vi "starSystemControl.vi"() -> ()   [LabVIEW 2021]
doc: "This example demonstrates how to call a Python function and pass doubles as arguments. It uses a python function to compute the sum of two doubles."
uses:
  <extravilib>/ChannelInstances/Tag-bool/Write With Abort.vi
  <extravilib>/ChannelInstances/Tag-bool/Read With Abort.vi
  <extravilib>/ChannelInstances/Tag-bool/Instantiate.vi
  <extravilib>/ChannelInstances/Tag-bool/EndpointRead.vi
  globalVariables.vi
  <extravilib>/ChannelInstances/Tag-bool/Endpoint.vi
  <extravilib>/ChannelInstances/Tag-bool.lvlib
  Copy of Kloehn V6 Series Folder/Copy of Kloehn V6 Series.lvlib
panel:
  out "armError":errorcluster
  in  "Motion":T1={"Top Speed (5000 sps) "=3000, "Start Speed (750 sps)"=750, "Stop Speed (750 sps)"=750, "Accel (17500 st/s^2)"=17500, "Decel (17500 st/s^2)"=17500, "Backlash Steps (100 steps)"=100}
  in  "syringeTotalVol":dbl=2.5
  in  "cDAQDirection_p1":tag="cDAQ1Mod1/port0/line0"
  in  "cDAQVoltage_p1":tag="cDAQ1Mod2/ao0"
  in  "voltage_p1":dbl=1.2 format="%#_3g"
  in  "rate_p1":dbl=2.6 format="%#_3g"
  in  "cDAQDirection_p2":tag="cDAQ1Mod1/port0/line1"
  in  "cDAQVoltage_p2":tag="cDAQ1Mod2/ao1"
  in  "locationPythonCode":path=path "C:/Users/coralProgram/Documents/armand/xArm-Python-SDK-master/main.py"
  in  "pythonVersion":dbl=3.9
  in  "robotName":string="a1"
  in  "pumpReverseVol":dbl=0.2
  in  "syringeReverseVol":dbl=0.2
  in  "voltage_p2":dbl=1.24 format="%#_3g"
  in  "rate_p2":dbl=2.09 caption="rate_p1" format="%#_3g"
  out "syringeError":errorcluster
  out "Response":string
  out "commandString":string
  in  "VISA Refnum in":refnum<visa-resource-name>="COM8"
  out "Gauge":dbl(knob) scale=0.0..7.0
  out "syringeState":dbl(slide)
  out "Position":dbl
  out "Busy":bool
  in  "Serial Configuration":cluster{"Baud Rate":u32, "Address":u16}={"Baud Rate"=9600, "Address"=1} {"Address" max=15 step=1}
  in  "VISA resource name":refnum<visa-resource-name>="COM7"
  in  "Array":dbl[][](array[numeric])=[[0.0, 10.0, 1.0], [10.0, 0.0, 1.0], [0.0, 10.0, 1.0], [10.0, 0.0, 1.0], [0.0, 10.0, 1.0], [10.0, 0.0, 1.0], [0.0, 10.0, 1.0], [10.0, 0.0, 1.0], [0.0, 10.0, 1.0], [10.0, 0.0, 1.0], [0.0, 10.0, 1.0], [10.0, 0.0, 1.0], [0.0, 10.0, 1.0], [10.0, 0.0, 1.0], [0.0, 10.0, 1.0], [10.0, 0.0, 1.0], [0.0, 10.0, 1.0], [10.0, 0.0, 1.0], [0.0, 10.0, 1.0], [10.0, 0.0, 1.0], [0.0, 10.0, 1.0], [10.0, 0.0, 1.0], [0.0, 10.0, 1.0], [10.0, 0.0, 1.0], [0.0, 10.0, 1.0], [10.0, 0.0, 1.0], [0.0, 10.0, 1.0], [10.0, 0.0, 1.0], [0.0, 10.0, 1.0], [10.0, 0.0, 1.0], [0.0, 10.0, 1.0], [10.0, 0.0, 1.0], [0.0, 10.0, 1.0], [10.0, 0.0, 1.0], [0.0, 10.0, 1.0], [10.0, 0.0, 1.0], [0.0, 10.0, 1.0], [10.0, 0.0, 1.0], [0.0, 10.0, 1.0], [10.0, 0.0, 1.0], [0.0, 10.0, 1.0], [10.0, 0.0, 1.0], [0.0, 10.0, 1.0], [10.0, 0.0, 1.0], [0.0, 10.0, 1.0], [10.0, 0.0, 1.0], [0.0, 10.0, 1.0], [10.0, 0.0, 1.0]]
  in  "stop_p1":bool caption="stop"
  out "position":dbl=45.0
  # "STAR System"
  # "Name"
  # "T1"
  # "Arm"
  # "Position"
  # "T2"
  # "T3"
  # "Python code location"
  # "Version"
  # "T4"
  # "T5"
  # "T6"
  # "Watchdog"
  # "Syringe error"
  # "T7"
  # "T8"
  # "Port"
  # "T9"
  # "T10"
  # "T11"
  # "Arm error"
  # "Command"
  # "T12"
  # "T13"
  # "Response"
  # "T14"
  # "T15"
  # "T16"
  # "T17"
  # "Syringe"
  # "T18"
  # "T19"
  # "Port"
  # "T20"
  # "Baud"
  # "T21"
  # "T22"
  # "Address"
  # "T23"
  # "T24"
  # "Total vol (mL)"
  # "T25"
  # "Reverse (mL)"
  # "T26"
  # "T27"
  # "Position"
  # "Busy"
  # "T28"
  # "T29"
  # "T30"
  # "T31"
  # "T32"
  # "T33"
  # "T34"
  # "T35"
  # "T36"
  # "T37"
  # "Pumps"
  # "Reverse (mL)"
  # "T38"
  # "T39"
  # "Pump 1"
  # "Pump 2"
  # "T40"
  # "Voltage"
  # "T41"
  # "T42"
  # "Rate (mL/S)"
  # "T43"
  # "T44"
  # "Voltage address"
  # "T45"
  # "T46"
  # "Direction address"
  # "T47"
  # "T48"
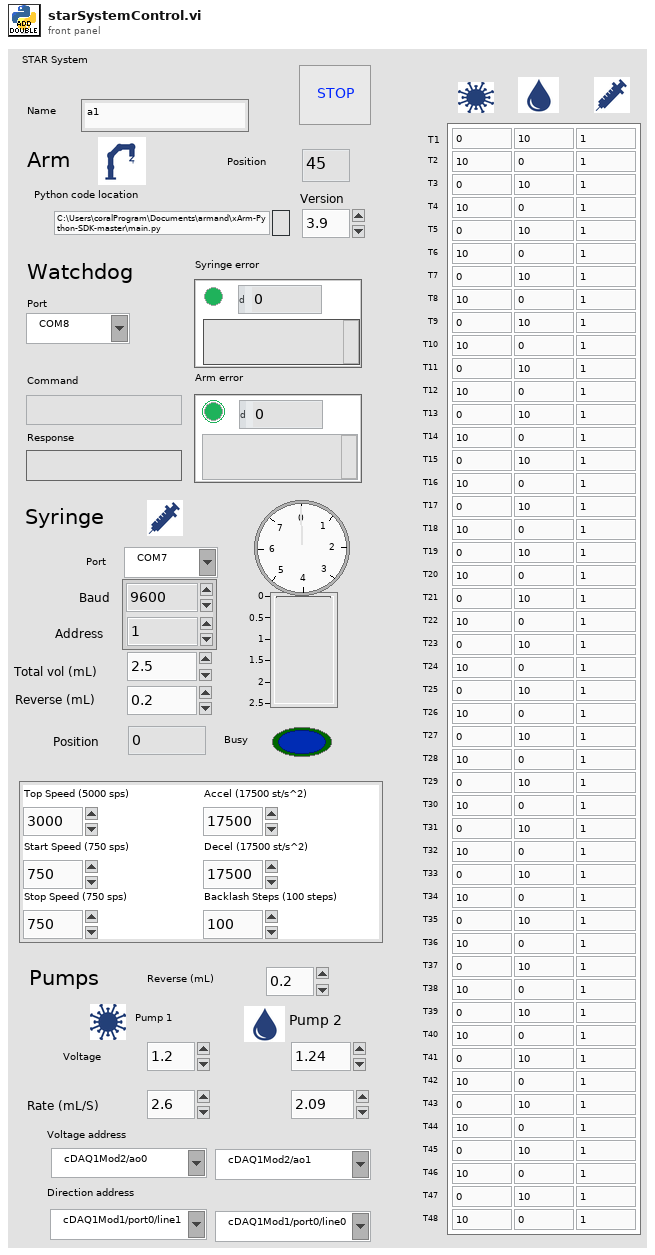
[diagram p1: front panel]
types:
  T1 = cluster{"Top Speed (5000 sps) ":i32, "Start Speed (750 sps)":i32, "Stop Speed (750 sps)":i32, "Accel (17500 st/s^2)":i32, "Decel (17500 st/s^2)":i32, "Backlash Steps (100 steps)":i32}
  T2 = typedef "Tag-bool.lvlib/))Channel.ctl" = refnum<queue>
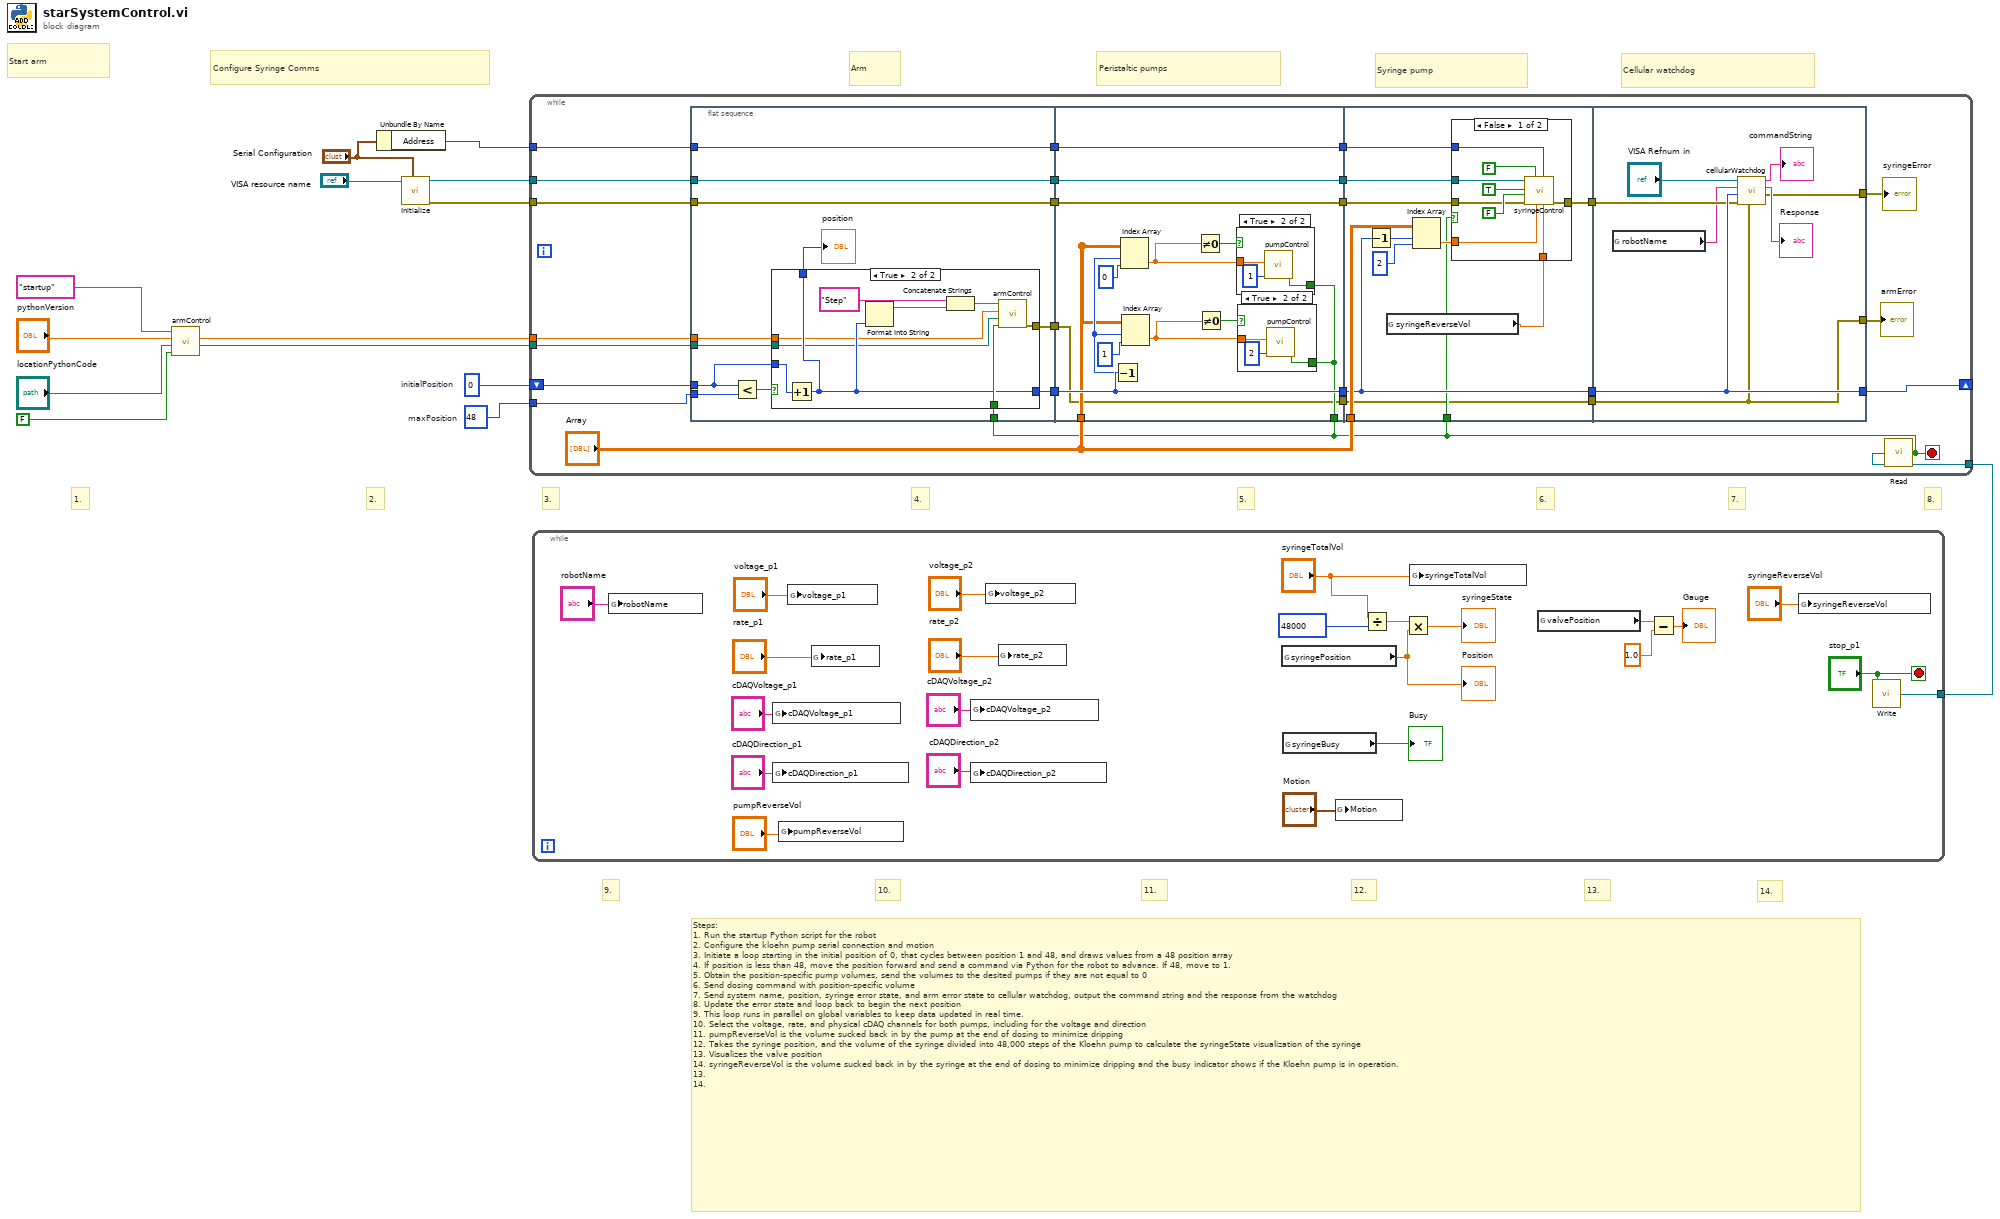
[diagram p0: block diagram]
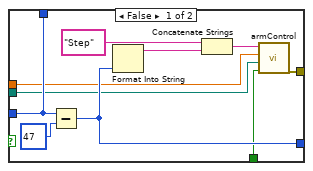
[diagram p2: hidden frame]
diagram:
  w12 = 48  # maxPosition
  w14 = 0  # initialPosition
  # "Start arm"
  # "Cellular watchdog"
  # "Syringe pump"
  # "Peristaltic pumps"
  # "Arm"
  # "14."
  # "Steps:\n1. Run the startup Python script for the robot\n2. Configure the kloehn pump serial connection and motion\n3. Initiate a loop starting in the initial position of 0, that cycles between position 1 and 48, and draws values from a 48 position array \n4. If position is less than 48, move the position forward and send a command via Python for the robot to advance. If 48, move to 1. \n5. Obtain the position-specific pump volumes, send the volumes to the desited pumps if they are not equal to 0\n6. Send dosing command with position-specific volume\n7. Send system name, position, syringe error state, and arm error state to cellular watchdog, output the command string and the response from the watchdog\n8. Update the error state and loop back to begin the next position\n9. This loop runs in parallel on global variables to keep data updated in real time. \n10. Select the voltage, rate, and physical cDAQ channels for both pumps, including for the voltage and direction\n11. pumpReverseVol is the volume sucked back in by the pump at the end of dosing to minimize dripping\n12. Takes the syringe position, and the volume of the syringe divided into 48,000 steps of the Kloehn pump to calculate the syringeState visualization of the syringe\n13. Visualizes the valve position\n14. syringeReverseVol is the volume sucked back in by the syringe at the end of dosing to minimize dripping and the busy indicator shows if the Kloehn pump is in operation.\n13.\n14."
  # "13."
  # "12."
  # "11."
  # "1."
  # "9."
  # "10."
  # "7."
  # "6."
  # "5."
  # "4."
  # "3."
  # "2."
  # "8."
  # "Configure Syringe Comms"
  n1 = call "armControl.vi"("Off"=FALSE ("buttonRefill"), "locationPythonCode"="locationPythonCode", "pythonVersionIn"="pythonVersion", "commandInput"="startup") -> ("locationPythonCodeOutput"=w3:path, "pythonVersionOut"=w4:dbl)  [unwired: 3 in, 2 out]
  n2 = Unbundle By Name("Serial Configuration") -> ("Address"=w6:u16)
  n3 = call "Initialize.vi"("Serial Configuration"="Serial Configuration", "VISA resource name"="VISA resource name") -> ("error out"=w8:errorcluster, "VISA resource name out"=w7:refnum<visa-resource-name>)  [unwired: 8 in]
  n4 = while {
    tunnel: [w37] -> w13
    stop <- "stop_p1" stop-if-true
    n5 = global write "globalVariables.vi" "robotName"("robotName") -> ()
    n6 = global write "globalVariables.vi" "cDAQVoltage_p1"("cDAQVoltage_p1") -> ()
    n7 = global write "globalVariables.vi" "cDAQDirection_p1"("cDAQDirection_p1") -> ()
    n8 = global write "globalVariables.vi" "pumpReverseVol"("pumpReverseVol") -> ()
    n9 = global write "globalVariables.vi" "voltage_p1"("voltage_p1") -> ()
    n10 = global write "globalVariables.vi" "rate_p1"("rate_p1") -> ()
    n11 = global write "globalVariables.vi" "cDAQVoltage_p2"("cDAQVoltage_p2") -> ()
    n12 = global write "globalVariables.vi" "cDAQDirection_p2"("cDAQDirection_p2") -> ()
    n13 = global write "globalVariables.vi" "voltage_p2"("voltage_p2") -> ()
    n14 = global write "globalVariables.vi" "rate_p2"("rate_p2") -> ()
    n15 = global read "globalVariables.vi" "syringePosition"() -> (w27:dbl)
    "Position" <- w27
    n16 = global read "globalVariables.vi" "syringeBusy"() -> (→"Busy":bool)
    n17 = global write "globalVariables.vi" "Motion"("Motion") -> ()
    n18 = Divide(x="syringeTotalVol", y=48000) -> (x/y=w34:dbl)
    n19 = Multiply(x=w34, y=w27) -> (x*y=→"syringeState":dbl)
    n20 = global write "globalVariables.vi" "syringeTotalVol"("syringeTotalVol") -> ()
    n21 = global read "globalVariables.vi" "valvePosition"() -> (w26:dbl)
    n22 = Subtract(x=w26, y=1.0) -> (x-y=→"Gauge":dbl)
    n23 = global write "globalVariables.vi" "syringeReverseVol"("syringeReverseVol") -> ()
    n24 = call <extravilib>:"Write.vi"("element"="stop_p1") -> ("channel"=w37:T2)  [unwired: 1 out]
  }
  n25 = while {
    shift-right: [w61] -> _
    shift-left: w14 -> [w44]
    tunnel: w13 -> [w63]
    tunnel: w12 -> [w62]
    tunnel: w8 -> [w59]
    tunnel: w7 -> [w48]
    tunnel: w6 -> [w47]
    tunnel: w4 -> [w43]
    tunnel: w3 -> [w42]
    stop <- w53 stop-if-true
    n26 = flat-sequence {
      tunnel: [w72] -> w57
      tunnel: w44 -> [w73]
      tunnel: w62 -> [w75]
      tunnel: w53 -> [w71]
      tunnel: [w70] -> w56
      tunnel: w59 -> [w70]
      tunnel: [w69] -> w49
      tunnel: w48 -> [w69]
      tunnel: w47 -> [w68]
      tunnel: [w68] -> w46
      tunnel: w43 -> [w66]
      tunnel: w42 -> [w65]
      tunnel: [w64] -> w38
      tunnel: [w108] -> w52
      tunnel: w57 -> [w108]
      tunnel: "Array" -> [w105]
      tunnel: w53 -> [w98]
      tunnel: [w103] -> w51
      tunnel: w56 -> [w103]
      tunnel: [w97] -> w50
      tunnel: w49 -> [w97]
      tunnel: w46 -> [w96]
      tunnel: [w96] -> w45
      tunnel: [w95] -> w39
      tunnel: w38 -> [w95]
      tunnel: w52 -> [w125]
      tunnel: "Array" -> [w126]
      tunnel: w53 -> [w121]
      tunnel: [w125] -> w55
      tunnel: [w120] -> w54
      tunnel: w51 -> [w119]
      tunnel: w50 -> [w118]
      tunnel: w45 -> [w117]
      tunnel: [w115] -> w40
      tunnel: w39 -> [w115]
      tunnel: [w144] -> w61
      tunnel: w55 -> [w144]
      tunnel: w54 -> [w140]
      tunnel: [w139] -> w58
      tunnel: [w137] -> w41
      tunnel: w40 -> [w137]
      frame #0 {
        n27 = Less?(x=w73, y=w75) -> (x < y?=w74:bool)
        n28 = case shown="True" w74 {
          tunnel: w73 -> [w79 w94]
          tunnel: [w82 w89] -> w72
          tunnel: w71 -> [w80 w90]
          tunnel: [w79 w89] -> w67
          tunnel: w66 -> [w78 w88]
          tunnel: w65 -> [w77 w87]
          tunnel: [w76 w86] -> w64
          frame False {
            n29 = Subtract(x=w79, y=47) -> (x-y=w82:i32)
            n30 = Format Into String(w82) -> (resulting string=w84:string)  [unwired: 3 in, 1 out]
            n31 = Concatenate Strings("Step", w84) -> (w85:string)
            n32 = call "armControl.vi"("Off"=w80, "locationPythonCode"=w77, "pythonVersionIn"=w78, "commandInput"=w85) -> ("armError"=w76:errorcluster)  [unwired: 3 in, 3 out]
          }
          frame True {
            n33 = Increment(x=w94) -> (x+1=w89:i32)
            n34 = Format Into String(w89) -> (resulting string=w92:string)  [unwired: 3 in, 1 out]
            n35 = Concatenate Strings("Step", w92) -> (w93:string)
            n36 = call "armControl.vi"("Off"=w90, "locationPythonCode"=w87, "pythonVersionIn"=w88, "commandInput"=w93) -> ("armError"=w86:errorcluster)  [unwired: 3 in, 3 out]
          }
        }
        "position" <- w67
      }
      frame #1 {
        n37 = Decrement(x=w108) -> (x-1=w107:i32)
        n38 = Index Array(array=w105, index (row)=w107, index (col)=0) -> (element=w101:dbl)
        n39 = Index Array(array=w105, index (row)=w107, index (col)=1) -> (element=w99:dbl)
        n40 = Not Equal To 0?(x=w101) -> (x != 0?=w102:bool)
        n41 = Not Equal To 0?(x=w99) -> (x != 0?=w100:bool)
        n42 = case shown="True" w102 {
          tunnel: w98 -> [_ w114]
          tunnel: w101 -> [_ w112]
          frame False {
          }
          frame True {
            n43 = call "pumpControl.vi"("OFF"=w114, "pump number"=1 ("Numeric"), "vol"=w112) -> ()  [unwired: 9 in]
          }
        }
        n44 = case shown="True" w100 {
          tunnel: w98 -> [_ w111]
          tunnel: w99 -> [_ w109]
          frame False {
          }
          frame True {
            n45 = call "pumpControl.vi"("OFF"=w111, "pump number"=2 ("Numeric"), "vol"=w109) -> ()  [unwired: 9 in]
          }
        }
      }
      frame #2 {
        n46 = Decrement(x=w125) -> (x-1=w124:i32)
        n47 = global read "globalVariables.vi" "syringeReverseVol"() -> (w116:dbl)
        n48 = Index Array(array=w126, index (row)=w124, index (col)=2) -> (element=w123:dbl)
        n49 = case shown="False" w121 {
          tunnel: w118 -> [w135 _]
          tunnel: w123 -> [w129 _]
          tunnel: [w128 w136] -> w120
          tunnel: w119 -> [w132 w136]
          tunnel: w117 -> [w131 _]
          tunnel: w116 -> [w127 _]
          frame False {
            n50 = call "syringeControl.vi"("syringeReverseVol"=w127, "Address"=w131, "volume(mL)"=w129, "buttonAspirate"=FALSE, "error in (no error)"=w132, "buttonRefill"=FALSE, "buttonDispense"=TRUE, "VISA Refnum in"=w135) -> ("error out"=w128:errorcluster)  [unwired: 2 in, 1 out]
          }
          frame True {
          }
        }
      }
      frame #3 {
        n51 = global read "globalVariables.vi" "robotName"() -> (w138:string)
        n52 = call "cellularWatchdog.vi"("armErrorIn"=w137, "syringeErrorIn"=w140, "robotPosition"=w144, "robotName"=w138, "VISA Refnum in"="VISA Refnum in") -> ("error out"=w139:errorcluster, "response"=→"Response":string, "concatenated string"=→"commandString":string)  [unwired: 4 in]
      }
    }
    n53 = call <extravilib>:"Read.vi"("channel"=w63) -> ("element"=w53:bool)  [unwired: 1 in, 1 out]
    "syringeError" <- w58
    "armError" <- w41
  }
